vi "Global.vi"() -> ()   [LabVIEW 2023, in "niUSRP Rx Core v1 FPGA.lvclass"]
uses:
  <instrlib>/niUSRP/Reference FPGA/Rx Core/niUSRP Rx Core v1 FPGA.lvclass
panel:
  out "enable":bool
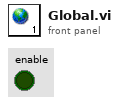
[diagram p1: front panel]
diagram:
